vi "WLAN_FrameAnalysis.vi"(8 "error in (no error)":errorcluster, 11 "input cluster":cluster{"t0":dbl, "dt":dbl, "Y":cdb[]}) -> (0 "error out":errorcluster, 1 "Constellation":cdb[](graph), 2 "Modulation parameter":T1, 3 "output bits":i8[](array[numeric]), 4 "Frequency offset":dbl, 5 "SIG valid?":bool)   [LabVIEW 2022 SP3]
panel:
  out "x+y":dbl
  out "Frequency offset(LTF)":dbl
  out "Frequency offset corrected signal 2":cluster{"t0":dbl, "dt":dbl, "Y":dbl[]}(graph)
  out "size(s) 3":i32
  out "size(s) 2":i32
  out "size(s)":i32
  out "Symbol numbers":i32
  out "encoded bit numbers":u32
  out "original bit numbers":u32
  out "Channel Esitimate":dbl[](graph)
  out "Frequency offset corrected signal":cluster{"t0":dbl, "dt":dbl, "Y":dbl[]}(graph)
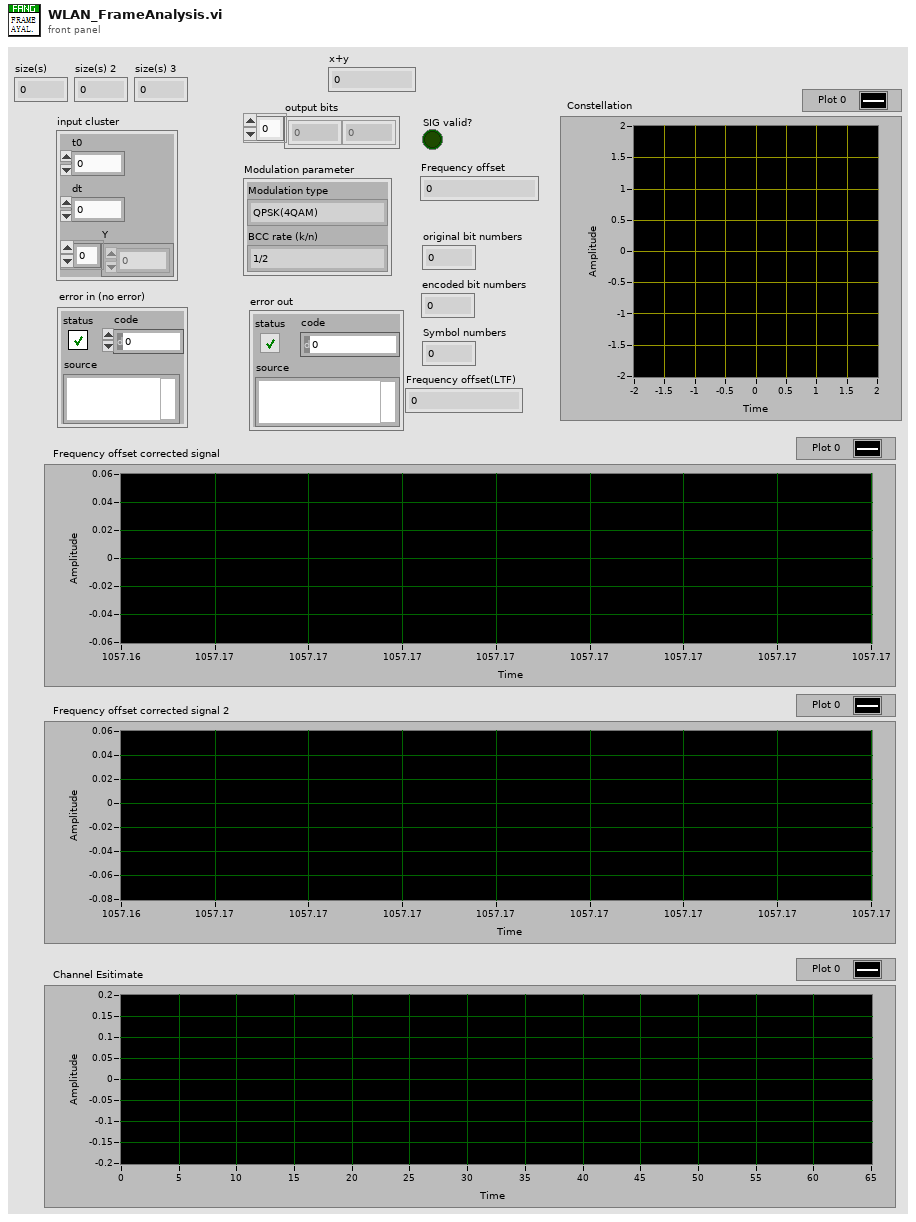
[diagram p1: front panel]
types:
  T1 = cluster{"Modulation type":enum16{"QPSK(4QAM)", "64QAM", "16QAM", "BPSK"}, "BCC rate (k/n)":enum16{"1/2", "2/3", "3/4"}}
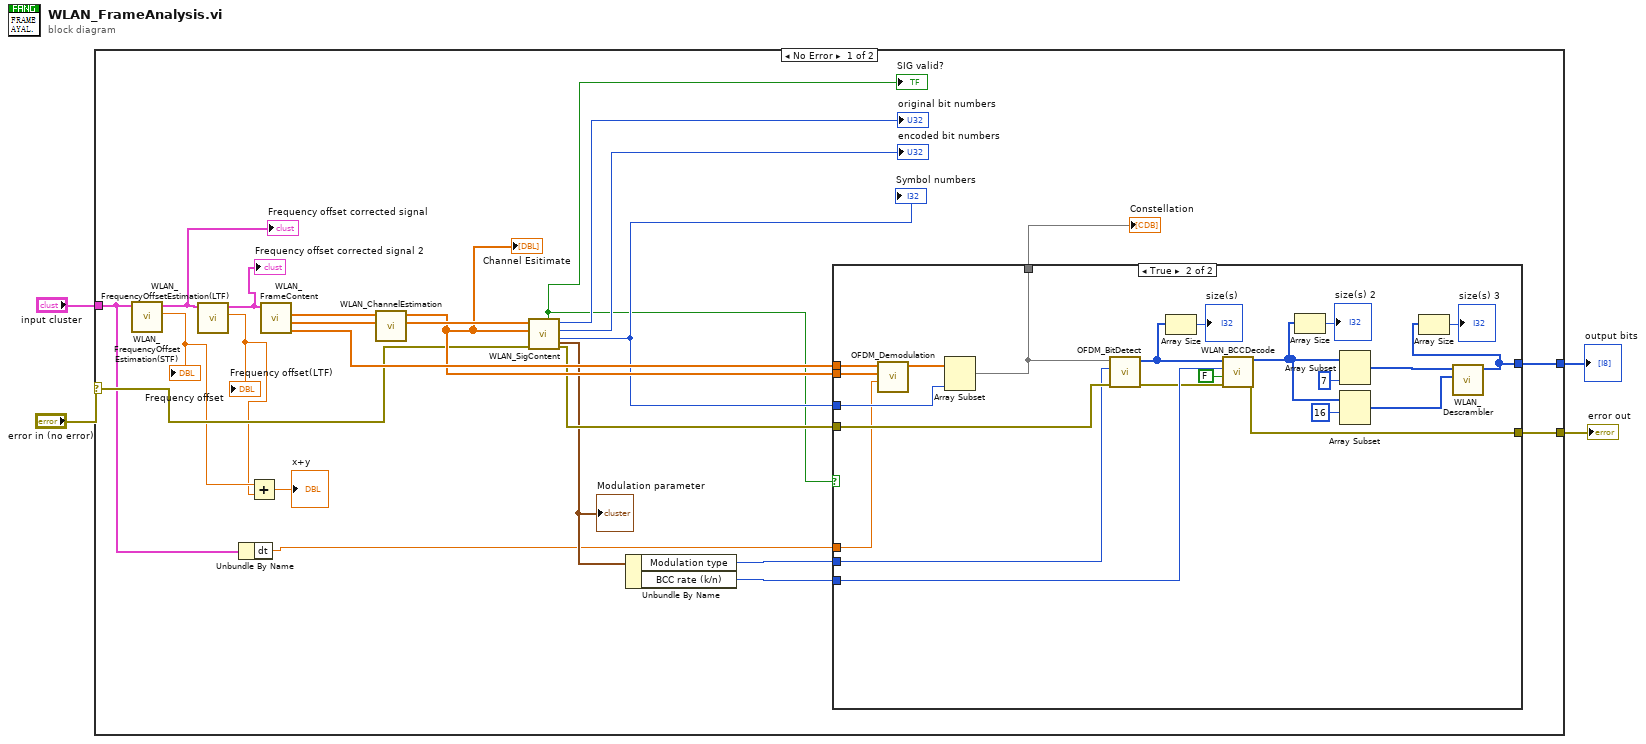
[diagram p0: block diagram]
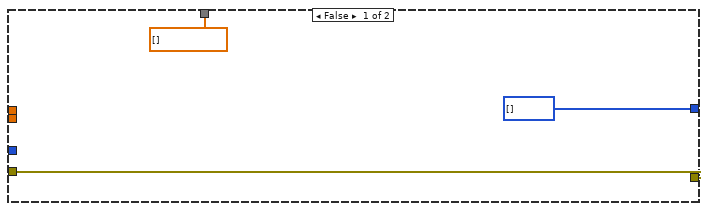
[diagram p2: hidden frame]
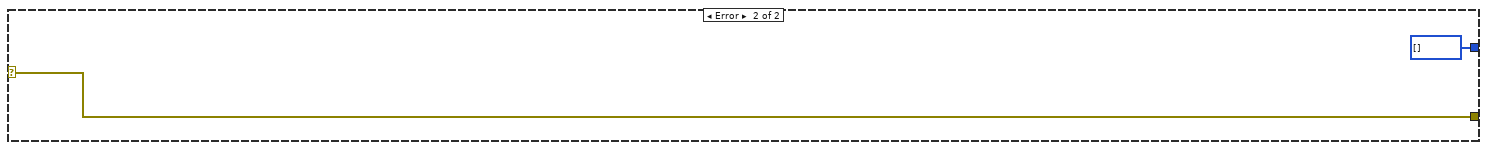
[diagram p3: hidden frame]
diagram:
  n1 = case shown="No Error" "error in (no error)" {
    selector: "error in (no error)" -> [w12 w53]
    tunnel: "input cluster" -> [w6 _]
    tunnel: [w19 w53] -> w3
    tunnel: [w18 i8[] [] ("scrambled bits")] -> w2
    frame No Error {
      n2 = call "WLAN_FrequencyOffsetEstimation(STF).vi"("output cluster"=w6) -> ("Frequency offset(STF)"=w10:dbl, "output cluster 2"=w11:cluster{"t0":dbl, "dt":dbl, "Y":cdb[]})  [unwired: 8 in]
      "Frequency offset corrected signal" <- w11
      "Frequency offset" <- w10
      n3 = call "WLAN_FrequencyOffsetEstimation(LTF).vi"("input cluster"=w11) -> ("Frequency offset(LTF)"=w9:dbl, "output cluster"=w7:cluster{"t0":dbl, "dt":dbl, "Y":cdb[]})  [unwired: 9 in]
      "Frequency offset corrected signal 2" <- w7
      "Frequency offset(LTF)" <- w9
      n4 = Unbundle By Name(w6) -> ("dt"=w5:dbl)
      n5 = Add(x=w10, y=w9) -> (x+y=→"x+y":dbl)
      n6 = call "WLAN_FrameContent.vi"("Input cluster"=w7) -> ("DATA"=w27:cdb[], "SIG"=w25:cdb[], "LTF"=w26:cdb[])  [unwired: 7 in, 1 out]
      n7 = call "WLAN_ChannelEstimation.vi"("LTF"=w26) -> ("Frequency estimation"=w24:cdb[])  [unwired: 10 in]
      "Channel Esitimate" <- w24
      n8 = call "WLAN_SigContent.vi"("error in (no error)"=w12, "Frequency channel estimation"=w24, "SIG"=w25) -> ("error out"=w23:errorcluster, "Symbol numbers"=w20:i32, "encoded bit numbers"=→"encoded bit numbers":u32, "original bit numbers"=→"original bit numbers":u32, "Modulation parameter"=w17:T1, "SIG valid?"=w13:bool)  [unwired: 3 in]
      "Modulation parameter" <- w17
      "Symbol numbers" <- w20
      "SIG valid?" <- w13
      n9 = Unbundle By Name(w17) -> ("Modulation type"=w16:enum16{"QPSK(4QAM)", "64QAM", "16QAM", "BPSK"}, "BCC rate (k/n)"=w15:enum16{"1/2", "2/3", "3/4"})
      n10 = case shown="True" w13 {
        tunnel: w27 -> [_ w52]
        tunnel: [w30 w44] -> w19
        tunnel: w24 -> [_ w50]
        tunnel: w23 -> [w30 w49]
        tunnel: w20 -> [_ w48]
        tunnel: w16 -> [_ w47]
        tunnel: [i8[] [] ("scrambled bits") w32] -> w18
        tunnel: w15 -> [_ w46]
        tunnel: [cdb[] [] w38] -> w14
        tunnel: w5 -> [_ w31]
        frame False {
        }
        frame True {
          n11 = call "OFDM_Demodulation.vi"("sampling period"=w31, "Frequency channel estimation"=w50, "Input sequence"=w52) -> ("Output sequence"=w51:cdb[])  [unwired: 8 in]
          n12 = Array Subset(array=w51, length=w48) -> (w38:cdb[])  [unwired: 1 in]
          n13 = call "OFDM_BitDetect.vi"("Input symbols"=w38, "Modulation type"=w47, "error in (no error)"=w49) -> ("Output bits"=w37:i8[], "error out"=w45:errorcluster)  [unwired: 6 in]
          n14 = Array Size(array=w37) -> (size(s)=→"size(s)":i32)
          n15 = call "WLAN_BCCDecode.vi"("error in (no error)"=w45, "need add zeros?"=FALSE, "BCC rate (k/n)"=w46, "input bit stream"=w37) -> ("error out"=w44:errorcluster, "output bit stream"=w34:i8[])  [unwired: 6 in]
          n16 = Array Size(array=w34) -> (size(s)=→"size(s) 2":i32)
          n17 = Array Subset(array=w34, length=7) -> (w40:i8[])  [unwired: 1 in]
          n18 = Array Subset(array=w34, index=16) -> (w41:i8[])  [unwired: 1 in]
          n19 = call "WLAN_Descrambler.vi"("scrambler initial bits"=w40, "data bits"=w41) -> ("scrambled bits"=w32:i8[])  [unwired: 7 in]
          n20 = Array Size(array=w32) -> (size(s)=→"size(s) 3":i32)
        }
      }
      "Constellation" <- w14
    }
    frame Error {
    }
  }
  "error out" <- w3
  "output bits" <- w2
